vi "PLC.IO.vi"(7 "Idx":i32, 8 "error in":errorcluster, 10 "DbRun":bool, 11 "Data_in":T1={"Status"={"Idx"=0, "ConnRef"=0, "State"=enum."Off", "LiveBitTimer"=timestamp(0 s since 1904-01-01)}, "Sets"={"Enable"=FALSE, "IP"="", "Rack"=0, "Slot"=0, "LifeBitTimer_s"=0.0, "DataBlockAddr_PCStatus"=0, "DataBlockAddr_PLCStatus"=1, "DataBlockAddr_PLCNewData"=[], "DataBlockSize_PLCNewData"=[], "DataBlockAddr_PLCChangeOver"=[], "DataBlockSize_PLCChangeOver"=[], "DataBlockAddr_PCChangeOver"=[], "DataBlockAddr_PLCCheckStatus"=[], "DataBlockSize_PLCCheckStatus"=[], "DataBlockAddr_PCCheckStatus"=[]}, "PCstatus"={"General"={"LifeBit"=FALSE, "DbRun"=FALSE}, "Stations"=[]}, "PLCstatus"={"General"={"LifeBit"=FALSE}, "Stations"=[]}}) -> (0 "error out":errorcluster, 3 "Data_out":T1={"Status"={"Idx"=0, "ConnRef"=0, "State"=enum."Off", "LiveBitTimer"=timestamp(0 s since 1904-01-01)}, "Sets"={"Enable"=FALSE, "IP"="", "Rack"=0, "Slot"=0, "LifeBitTimer_s"=0.0, "DataBlockAddr_PCStatus"=0, "DataBlockAddr_PLCStatus"=1, "DataBlockAddr_PLCNewData"=[], "DataBlockSize_PLCNewData"=[], "DataBlockAddr_PLCChangeOver"=[], "DataBlockSize_PLCChangeOver"=[], "DataBlockAddr_PCChangeOver"=[], "DataBlockAddr_PLCCheckStatus"=[], "DataBlockSize_PLCCheckStatus"=[], "DataBlockAddr_PCCheckStatus"=[]}, "PCstatus"={"General"={"LifeBit"=FALSE, "DbRun"=FALSE}, "Stations"=[]}, "PLCstatus"={"General"={"LifeBit"=FALSE}, "Stations"=[]}})   [LabVIEW 2016]
doc: "Read data block from PLC to PC and write data block from PC to PLC. Control live bit of PC\n\nWabco 2017 All right reserved\nAuthor: maciej.szupienko@wabco-auto.com"
uses:
  PLC.Data.ctl
  PLC.Data.Status.ctl
  PLC.State.ctl
  PLC.Data.Sets.ctl
  LowLevel/PLC.DataBlock.PCstatus.ctl
  LowLevel/PLC.DataBlock.PCstatus.General.ctl
  LowLevel/PLC.DataBlock.PCstatus.Station.ctl
  LowLevel/PLC.DataBlock.PLCstatus.ctl
  LowLevel/PLC.DataBlock.PLCstatus.General.ctl
  LowLevel/PLC.DataBlock.PLCstatus.Station.ctl
  Tools/EventLog/EventLog.EventSource.ctl
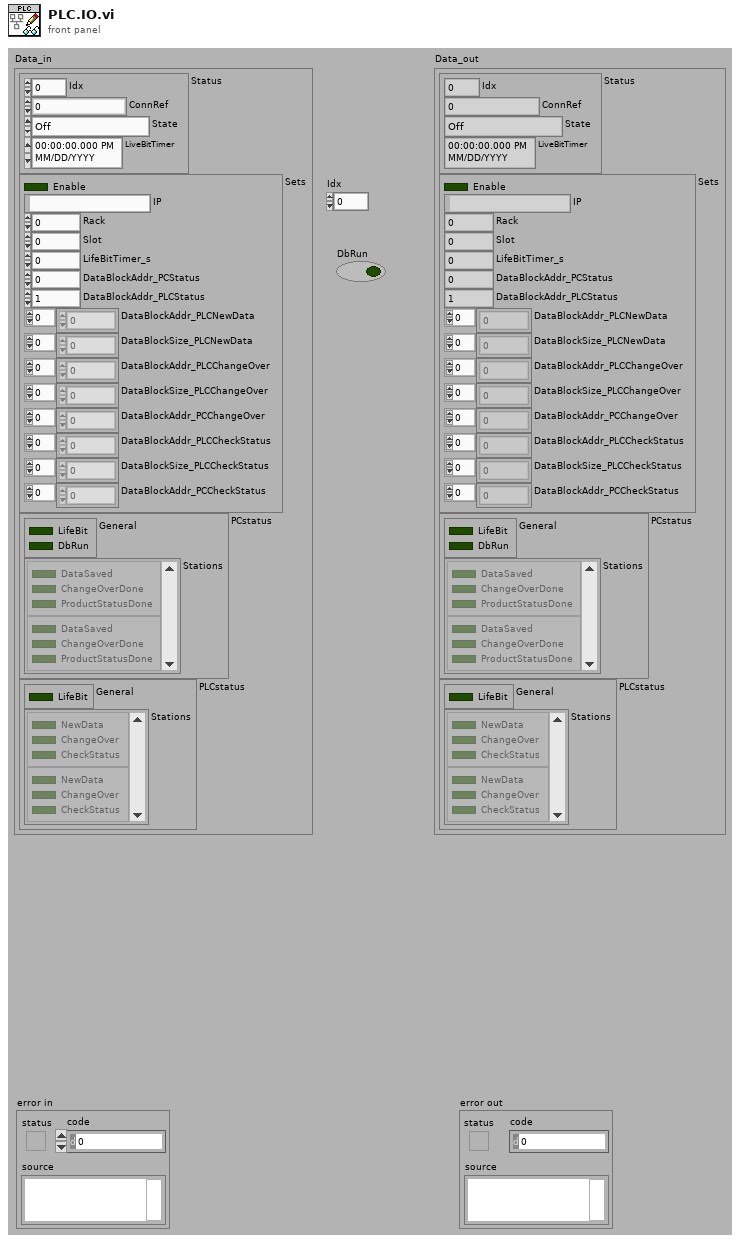
[diagram p1: front panel]
types:
  T1 = typedef "PLC.Data.ctl" = cluster{"Status":T2, "Sets":T4, "PCstatus":T5, "PLCstatus":T8}
  T2 = typedef "PLC.Data.Status.ctl" = cluster{"Idx":i32, "ConnRef":u64, "State":T3, "LiveBitTimer":timestamp}
  T3 = typedef "PLC.State.ctl" = enum32{"Off", "Error", "Idle", "Run"}
  T4 = typedef "PLC.Data.Sets.ctl" = cluster{"Enable":bool, "IP":string, "Rack":i32, "Slot":i32, "LifeBitTimer_s":dbl, "DataBlockAddr_PCStatus":i32, "DataBlockAddr_PLCStatus":i32, "DataBlockAddr_PLCNewData":i32[], "DataBlockSize_PLCNewData":i32[], "DataBlockAddr_PLCChangeOver":i32[], "DataBlockSize_PLCChangeOver":i32[], "DataBlockAddr_PCChangeOver":i32[], "DataBlockAddr_PLCCheckStatus":i32[], "DataBlockSize_PLCCheckStatus":i32[], "DataBlockAddr_PCCheckStatus":i32[]}
  T5 = typedef "PLC.DataBlock.PCstatus.ctl" = cluster{"General":T6, "Stations":T7[]}
  T6 = typedef "PLC.DataBlock.PCstatus.General.ctl" = cluster{"LifeBit":bool, "DbRun":bool}
  T7 = typedef "PLC.DataBlock.PCstatus.Station.ctl" = cluster{"DataSaved":bool, "ChangeOverDone":bool, "ProductStatusDone":bool}
  T8 = typedef "PLC.DataBlock.PLCstatus.ctl" = cluster{"General":T9, "Stations":T10[]}
  T9 = typedef "PLC.DataBlock.PLCstatus.General.ctl" = cluster{"LifeBit":bool}
  T10 = typedef "PLC.DataBlock.PLCstatus.Station.ctl" = cluster{"NewData":bool, "ChangeOver":bool, "CheckStatus":bool}
  T11 = typedef "EventLog.EventSource.ctl" = enum16{"All", "Gui", "Cache", "PLC1", "PLC2", "PLC3", "DB", "DB01", "DB02", "DB03", "DB04", "DB05", "DB06", "DB07", "DB08", "DB09", "DB10", "DB11", "DB12", "DB13", "DB14", "DB15", "DB16"}
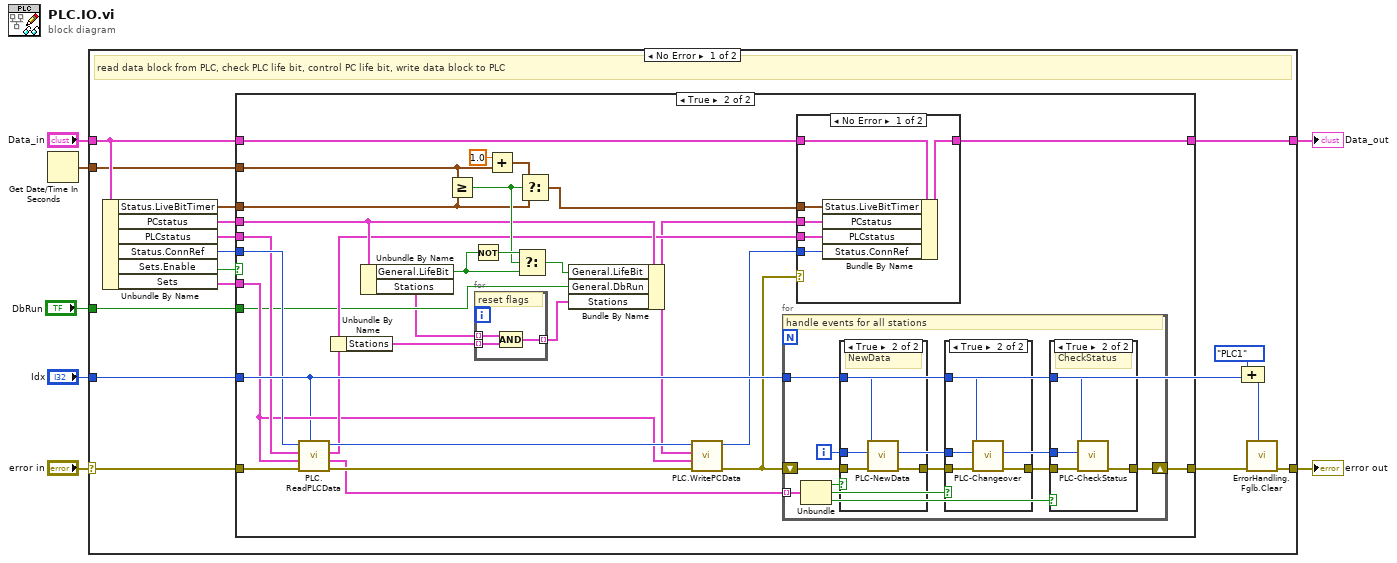
[diagram p0: block diagram]
diagram:
  n1 = Get Date/Time In Seconds() -> (seconds since 1Jan1904=w3:timestamp)
  n2 = case shown="No Error" "error in" {
    selector: "error in" -> [w20 w91]
    tunnel: [w22 w91] -> w4
    tunnel: "Data_in" -> [w21 w90]
    tunnel: [w23 w90] -> w6
    tunnel: w3 -> [w19 _]
    tunnel: "Idx" -> [w11 _]
    tunnel: "DbRun" -> [w8 _]
    frame No Error {
      # "read data block from PLC, check PLC life bit, control PC life bit, write data block to PLC"
      n3 = Unbundle By Name(w21) -> ("Status.LiveBitTimer"=w18:timestamp, "PCstatus"=w17:T5, "PLCstatus"=w14:T8, "Status.ConnRef"=w16:u64, "Sets.Enable"=w13:bool, "Sets"=w12:T4)
      n4 = case shown="True" w13 {
        tunnel: [w25 w54] -> w23
        tunnel: w21 -> [w25 w53]
        tunnel: w20 -> [w24 w39]
        tunnel: w19 -> [_ w50]
        tunnel: w18 -> [_ w49]
        tunnel: w17 -> [_ w48]
        tunnel: w16 -> [_ w41]
        tunnel: [w24 w45] -> w15
        tunnel: w14 -> [_ w40]
        tunnel: w12 -> [_ w35]
        tunnel: w11 -> [_ w34]
        tunnel: w8 -> [_ w30]
        frame False {
        }
        frame True {
          n5 = call "PLC.ReadPLCData.vi"("Idx"=w34, "error in (no error)"=w39, "Sets"=w35, "PLCdata in"=w40, "Ref in"=w41) -> ("error out"=w36:errorcluster, "Events"=w31:T10[], "PLCdata out"=w37:T8, "Ref out"=w38:u64)  [unwired: 3 in]
          n6 = Unbundle By Name(w37) -> ("Stations"=w47:T10[])
          n7 = Unbundle By Name(w48) -> ("General.LifeBit"=w46:bool, "Stations"=w29:T7[])
          n8 = Greater Or Equal?(x=w50, y=w49) -> (x >= y?=w51:bool)
          n9 = Not(x=w46) -> (.not. x?=w52:bool)
          n10 = for {
            tunnel: w47 -> [w81] mode=indexing
            tunnel: w29 -> [w82] mode=indexing
            tunnel: [w80] -> w27 mode=indexing
            # "reset flags"
            n11 = Compound Arithmetic op=AND(w82, w81) -> (w80:T7)
          }
          n12 = Add(x=1.0 ("y"), y=w50) -> (x+y=w44:timestamp)
          n13 = Select(t=w52, s=w51, f=w46) -> (s? t:f=w26:bool)
          n14 = Select(t=w44, s=w51, f=w49) -> (s? t:f=w42:timestamp)
          n15 = Bundle By Name(cluster=w48, "General.LifeBit"=w26, "General.DbRun"=w30, "Stations"=w27) -> (w28:T5)
          n16 = call "PLC.WritePCData.vi"("error in (no error)"=w36, "Sets"=w35, "PCdata in"=w28, "Ref in"=w38) -> ("error out"=w32:errorcluster, "Ref out"=w33:u64)  [unwired: 5 in, 1 out]
          n17 = for {
            tunnel: w34 -> [w56]
            shift-right: [w55] -> w45
            shift-left: w32 -> [w64]
            tunnel: w31 -> [w63] mode=indexing
            i -> [w57]
            # "handle events for all stations"
            n18 = Unbundle(w63) -> ("NewData"=w62:bool, "ChangeOver"=w61:bool, "CheckStatus"=w58:bool)
            n19 = case shown="True" w62 {
              tunnel: w64 -> [w75 w79]
              tunnel: [w75 w78] -> w60
              tunnel: w56 -> [_ w77]
              tunnel: w57 -> [_ w76]
              frame False {
              }
              frame True {
                # "NewData"
                n20 = call "PLC-NewData.vi"("error in"=w79, "Slot"=w76, "Idx"=w77) -> ("error out"=w78:errorcluster)  [unwired: 8 in]
              }
            }
            n21 = case shown="True" w61 {
              tunnel: w60 -> [w70 w71]
              tunnel: [w70 w74] -> w59
              tunnel: w56 -> [_ w73]
              tunnel: w57 -> [_ w72]
              frame False {
                # "ChangeOver"
              }
              frame True {
                n22 = call "PLC-Changeover.vi"("error in"=w71, "Slot"=w72, "Idx"=w73) -> ("error out"=w74:errorcluster)  [unwired: 8 in]
              }
            }
            n23 = case shown="True" w58 {
              tunnel: w59 -> [w65 w66]
              tunnel: [w65 w69] -> w55
              tunnel: w56 -> [_ w68]
              tunnel: w57 -> [_ w67]
              frame False {
              }
              frame True {
                # "CheckStatus"
                n24 = call "PLC-CheckStatus.vi"("error in"=w66, "Slot"=w67, "Idx"=w68) -> ("error out"=w69:errorcluster)  [unwired: 8 in]
              }
            }
          }
          n25 = case shown="No Error" w32 {
            tunnel: [w88 w89] -> w54
            tunnel: w53 -> [w87 w89]
            tunnel: w28 -> [w86 _]
            tunnel: w37 -> [w85 _]
            tunnel: w42 -> [w84 _]
            tunnel: w33 -> [w83 _]
            frame No Error {
              n26 = Bundle By Name(cluster=w87, "Status.LiveBitTimer"=w84, "PCstatus"=w86, "PLCstatus"=w85, "Status.ConnRef"=w83) -> (w88:T1)
            }
            frame Error {
            }
          }
        }
      }
      n27 = Compound Arithmetic op=ADD(EventLog.EventSource."PLC1" ("Event source"), w11) -> (w9:i32)
      n28 = call "ErrorHandling.Fglb.Clear.vi"("Event source"=w9, "error in (no error)"=w15) -> ("error out"=w22:errorcluster)  [unwired: 9 in]
    }
    frame Error {
    }
  }
  "error out" <- w4
  "Data_out" <- w6
